vi "CheckIfValid.vi"(7 "check all internal refs? (F)":bool, 8 "error in":errorcluster, 11 "error reporter in":refnum<class "ErrorReporter.lvclass">) -> (0 "error out":errorcluster, 2 "valid?":bool, 3 "error reporter out":refnum<class "ErrorReporter.lvclass">)   [LabVIEW 2014, in "CLM_ErrorHandler.lvlib" / "ErrorReporter.lvclass"]
uses:
  ErrorReporter.lvclass
  ErrorReporter.lvclass/ErrorReporter.ctl
  <vilib>/CLM/LocalMessenger/PriorityLocalMessage/CLM_PriorityLocalMessage.lvclass
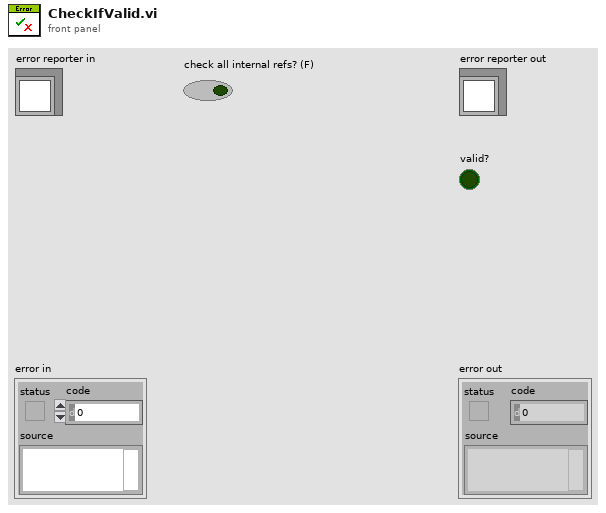
[diagram p1: front panel]
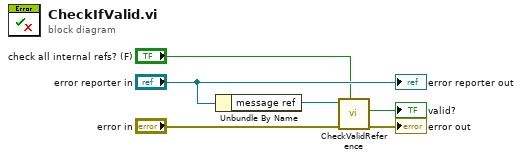
[diagram p0: block diagram]
diagram:
  n1 = Unbundle By Name("error reporter in") -> ("message ref"=w5:refnum<class "CLM_PriorityLocalMessage.lvclass">)
  n2 = call <vilib>:"CheckValidReference.vi"("check all queues? (F)"="check all internal refs? (F)", "error in"="error in", "message ref in"=w5) -> ("error out"=→"error out":errorcluster, "valid?"=→"valid?":bool)  [unwired: 6 in, 1 out]
  "error reporter out" <- "error reporter in"
